vi "U.vi"() -> ()   [LabVIEW 2014]
uses:
  <vilib>/regexp/Match Regular Expression.xnode
panel:
  out "Array":string[](array[string])
  out "error out":errorcluster caption="错误输出"
  in  "error in (no error)":errorcluster caption="错误输入（无错误）"
  in  "String":string
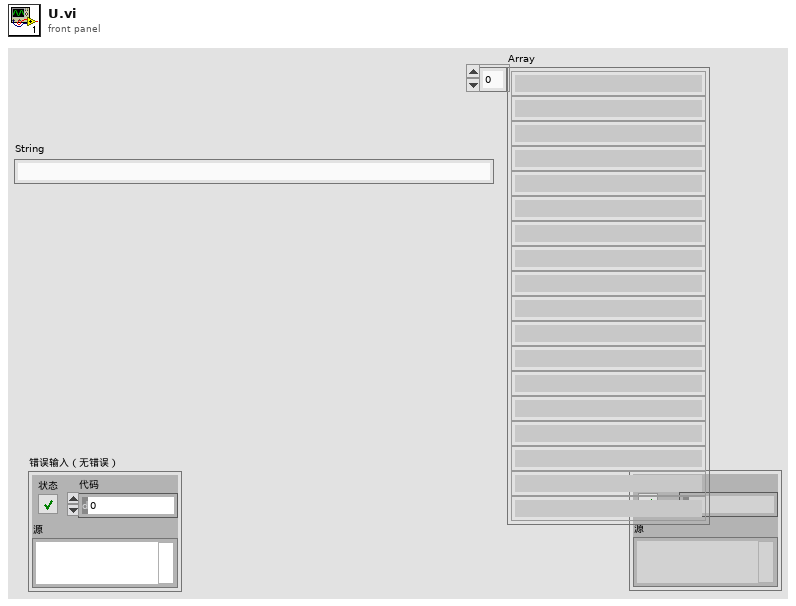
[diagram p1: front panel]
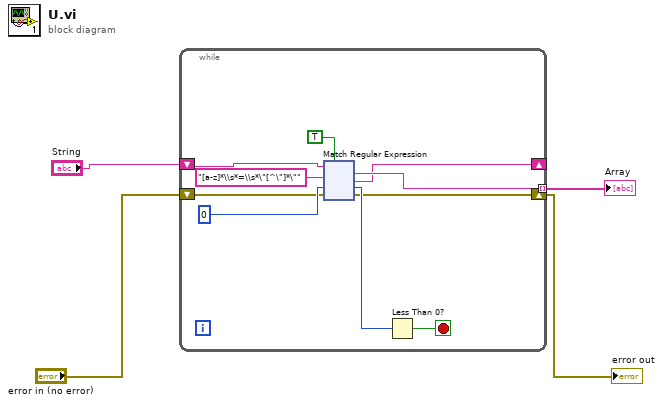
[diagram p0: block diagram]
diagram:
  n1 = while {
    shift-right: [w8] -> _
    shift-left: "String" -> [w14]
    tunnel: [w10] -> w3 mode=indexing
    shift-right: [w5] -> w1
    shift-left: "error in (no error)" -> [w6]
    stop <- w11 stop-if-true
    n2 = xnode "Match Regular Expression"("input string"=w14, "regular expression"="[a-z]*\\s*=\\s*\"[^\"]*\"", "offset (0)"=0, "error in"=w6, "ignore case? (F)"=TRUE) -> ("whole match"=w10:string, "after match"=w8:string, "offset past match"=w9:i32, "error out"=w5:errorcluster)  [unwired: 1 in, 1 out]
    n3 = Less Than 0?(x=w9) -> (x < 0?=w11:bool)
  }
  "error out" <- w1
  "Array" <- w3
